vi "Event Wait Data.vi"(8 "error in (no error)":errorcluster, 11 "Event DVR in":refnum<data-value>) -> (0 "error out":errorcluster, 2 "Data out":refnum<data-value>, 3 "Event DVR out":refnum<data-value>)   [LabVIEW 2012, in "MDSplus.lvlib"]
doc: "Return data received last."
uses:
  <vilib>/MDSplus/Library/MDSplus.lvlib
  <vilib>/MDSplus/Classes/Event_Class/Event.lvclass
  <vilib>/MDSplus/Classes/Data_Class/Data.lvclass
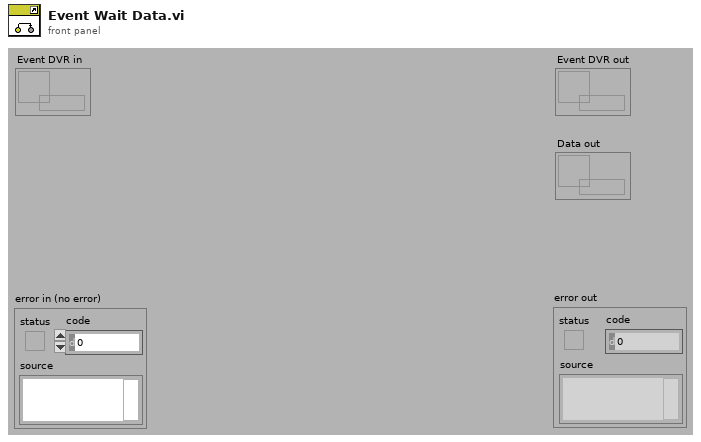
[diagram p1: front panel]
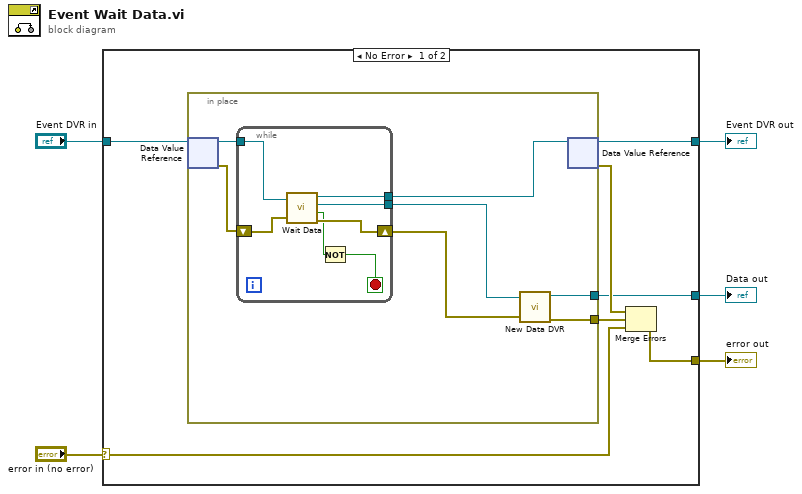
[diagram p0: block diagram]
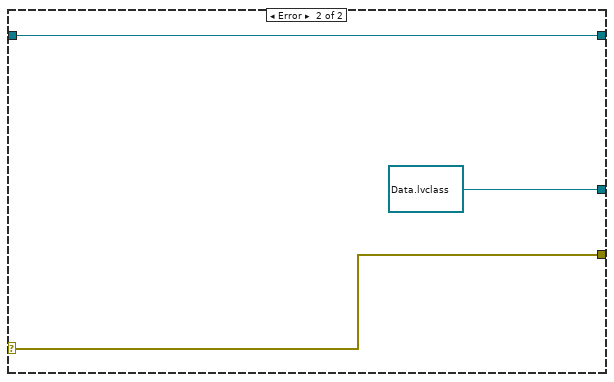
[diagram p2: hidden frame]
diagram:
  n1 = case shown="No Error" "error in (no error)" {
    selector: "error in (no error)" -> [w11 w29]
    tunnel: "Event DVR in" -> [w12 w28]
    tunnel: [w8 w29] -> w5
    tunnel: [w9 w28] -> w2
    tunnel: [w6 refnum<data-value> refnum ("Data DVR")] -> w1
    frame No Error {
      n2 = in-place {
        in-place-border: [w19] -> w6
        in-place-border: [w18] -> w7
        n3 = in-place-dvr #1(w12) -> (w17:refnum<class "Event.lvclass">, w14:errorcluster)
        n4 = while {
          tunnel: w17 -> [w26]
          tunnel: [w25] -> w16
          tunnel: [w24] -> w15
          shift-right: [w22] -> w13
          shift-left: w14 -> [w23]
          stop <- w20 stop-if-true
          n5 = call-dynamic "Wait Data.vi"("error in (no error)"=w23, "Event in"=w26) -> ("error out"=w22:errorcluster, "Timeout Occurred"=w21:bool, "Data out"=w25:refnum<class "Data.lvclass">, "Event out"=w24:refnum<class "Event.lvclass">)  [unwired: 6 in]
          n6 = Not(x=w21) -> (.not. x?=w20:bool)
        }
        n7 = call <vilib>:"New Data DVR.vi"("error in (no error)"=w13, "Data in"=w16) -> ("error out"=w18:errorcluster, "Data DVR out"=w19:refnum<data-value>)  [unwired: 8 in]
        n8 = in-place-dvr #1(w15) -> (w9:refnum<data-value>, w10:errorcluster)
      }
      n9 = Merge Errors(w10, w7, w11) -> (w8:errorcluster)
    }
    frame Error {
    }
  }
  "error out" <- w5
  "Event DVR out" <- w2
  "Data out" <- w1
